vi "CheckAbnormal.vi"(6 "Status":refnum<vi>, 9 "Known Found?":bool, 10 "Filenames":string[](array[string])) -> (1 "Ignore":bool, 2 "Filenames out":string[](array[string]))   [LabVIEW 2022 SP3]
uses:
  <vilib>/Analysis/NI_AALBase.lvlib
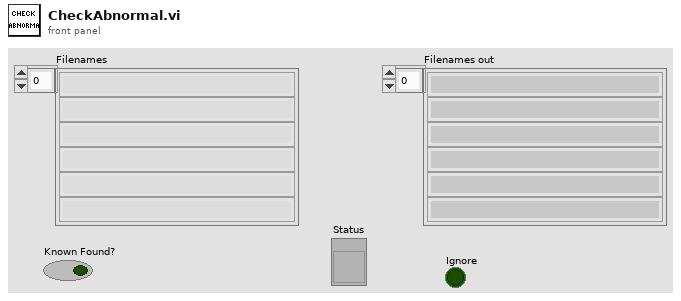
[diagram p1: front panel]
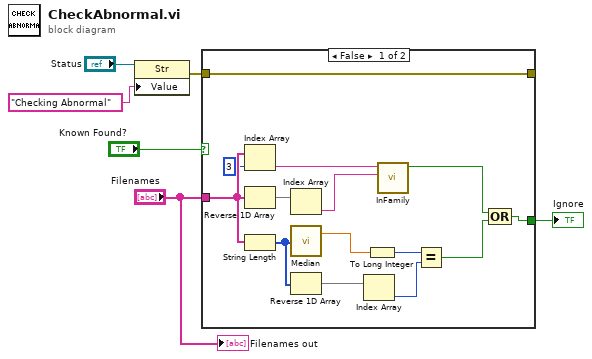
[diagram p0: block diagram]
diagram:
  n1 = property class="Str"(reference="Status", "Value"="Checking Abnormal") -> (error out=w1:errorcluster)  [unwired: 1 in, 1 out]
  n2 = case shown="False" "Known Found?" {
    tunnel: "Filenames" -> [w12 _]
    tunnel: [w13 _] -> w5
    tunnel: w1 -> [w15 w21]
    tunnel: [w15 w21] -> _
    frame False {
      n3 = Index Array(array=w12, index=3) -> (element=w10:string)
      n4 = Reverse 1D Array(array=w12) -> (reversed array=w16:string[])
      n5 = String Length(string=w12) -> (length=w20:i32[])
      n6 = Index Array(array=w16) -> (element=w9:string)  [unwired: 1 in]
      n7 = call <vilib>:"Median.vi"("X"=w20) -> ("median"=w14:dbl)  [unwired: 1 out]
      n8 = Reverse 1D Array(array=w20) -> (reversed array=w18:i32[])
      n9 = Index Array(array=w18) -> (element=w17:i32)  [unwired: 1 in]
      n10 = To Long Integer(number=w14) -> (32bit integer=w19:i32)
      n11 = call "InFamily.vi"("String 2"=w9, "String 1"=w10) -> ("Family?"=w8:bool)  [unwired: 9 in]
      n12 = Equal?(x=w19, y=w17) -> (x = y?=w7:bool)
      n13 = Compound Arithmetic op=OR(w8, w7) -> (w13:bool)
    }
    frame True {
    }
  }
  "Ignore" <- w5
  "Filenames out" <- "Filenames"
